vi "RecordFC.vi"(7 "FC-Data":string[][](array[string]), 8 "Latching":bool, 9 "RecordFCdata":bool, 10 "error in (no error)":errorcluster caption="Fehler (Eingang, kein Fehler)", 11 "MultiWii Data Cluster 2":refnum<vi>) -> (2 "error out":errorcluster caption="Fehler (Ausgang)", 5 "FC-Data OUT":string[][](array[string]))   [LabVIEW 2017]
uses:
  IMU_Functions/IMU_Data_Cluster.ctl
  <vilib>/Utility/file.llb/Write To Spreadsheet File (string).vi
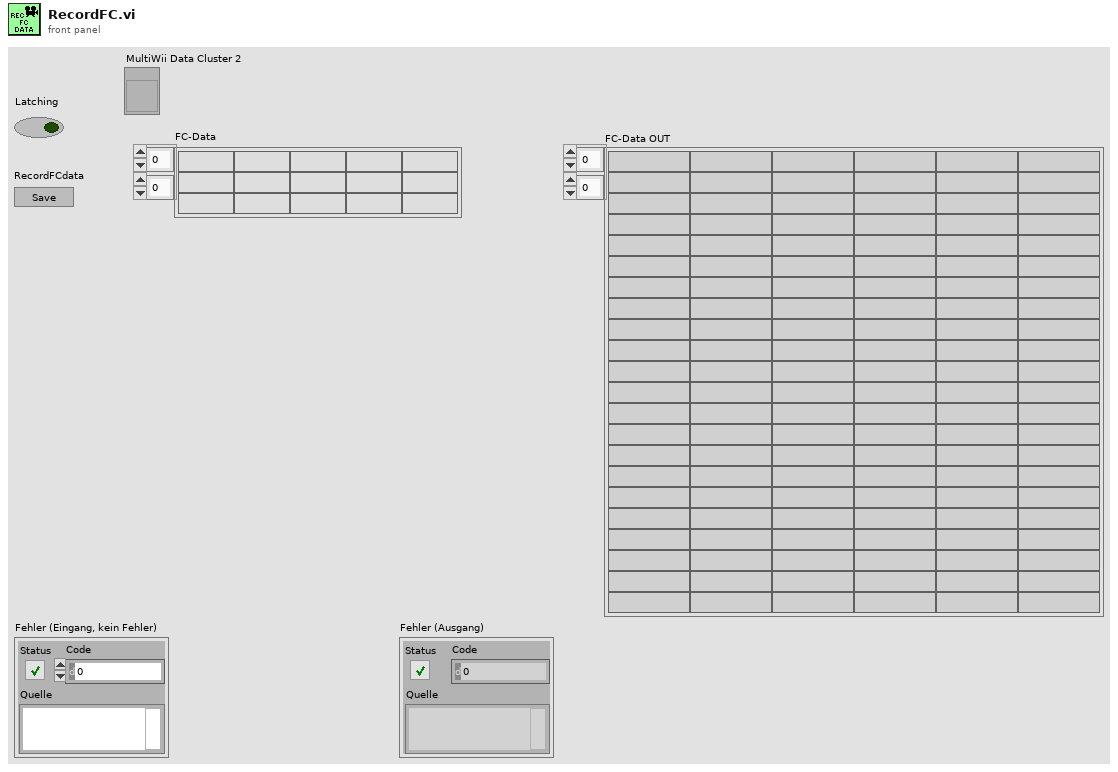
[diagram p1: front panel]
types:
  T1 = typedef "IMU_Data_Cluster.ctl" = cluster{"Firmware Revision":string, "Multitype Name":string, "Cycle Time":u16, "I²C Error Count":u16, "ACC present":bool, "Baro present":bool, "Mag Present":bool, "GPS present":bool, "Sonar present":bool, "Acc X axis (Roll)":dbl, "Acc Y axis (Pitch)":dbl, "Acc Z axis (Yaw)":dbl, "Gyro X axis (Roll)":dbl, "Gyro Y axis (Pitch)":dbl, "Gyro Z axis (Yaw)":dbl, "Mag X axis (Roll)":dbl, "Mag Y axis (Pitch)":dbl, "Mag Z axis (Yaw)":dbl, "X angle (Roll)":dbl, "Y angle (Pitch)":dbl, "Heading [°]":dbl, "Altitude [m]":dbl, "Vario":dbl, "GPS_Fix":u8, "GPS_NumSat":u8, "GPS_coord[LAT]":dbl, "GPS_coord[LON]":dbl, "GPS_Altitude":dbl, "GPS_Speed over Ground":dbl, "GPS_Ground Course":dbl, "Baro P [mbara]":dbl, "Baro T [°C]":dbl, "Altitude abs [m]":dbl}
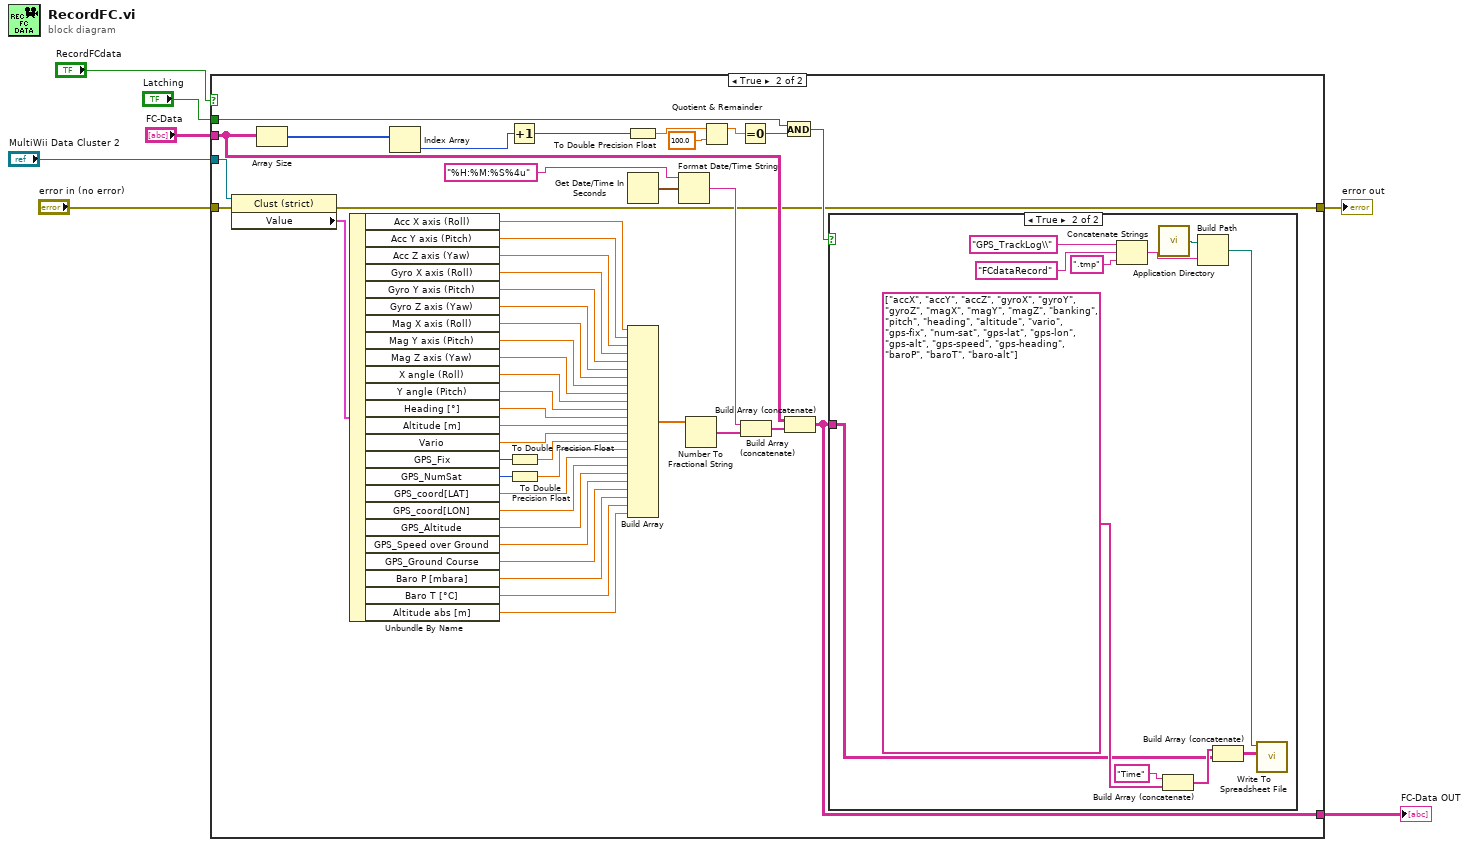
[diagram p0: block diagram]
diagram:
  n1 = case shown="True" "RecordFCdata" {
    tunnel: "FC-Data" -> [w9 w28]
    tunnel: [w9 w22] -> w5
    tunnel: "Latching" -> [_ w20]
    tunnel: "MultiWii Data Cluster 2" -> [_ w13]
    tunnel: "error in (no error)" -> [w8 w11]
    tunnel: [w8 w10] -> w1
    frame False {
    }
    frame True {
      n2 = property class="Clust (strict)"(reference=w13, error in=w11) -> (error out=w10:errorcluster, "Value"=w12:T1)  [unwired: 1 out]
      n3 = Array Size(array=w28) -> (size(s)=w29:i32[])
      n4 = Unbundle By Name(w12) -> ("Acc X axis (Roll)"=w56:dbl, "Acc Y axis (Pitch)"=w55:dbl, "Acc Z axis (Yaw)"=w54:dbl, "Gyro X axis (Roll)"=w53:dbl, "Gyro Y axis (Pitch)"=w52:dbl, "Gyro Z axis (Yaw)"=w51:dbl, "Mag X axis (Roll)"=w50:dbl, "Mag Y axis (Pitch)"=w49:dbl, "Mag Z axis (Yaw)"=w48:dbl, "X angle (Roll)"=w47:dbl, "Y angle (Pitch)"=w46:dbl, "Heading [°]"=w45:dbl, "Altitude [m]"=w43:dbl, "Vario"=w42:dbl, "GPS_Fix"=w41:u8, "GPS_NumSat"=w40:u8, "GPS_coord[LAT]"=w39:dbl, "GPS_coord[LON]"=w38:dbl, "GPS_Altitude"=w37:dbl, "GPS_Speed over Ground"=w36:dbl, "GPS_Ground Course"=w33:dbl, "Baro P [mbara]"=w32:dbl, "Baro T [°C]"=w31:dbl, "Altitude abs [m]"=w30:dbl)
      n5 = Index Array(array=w29) -> (element=w27:i32)  [unwired: 1 in]
      n6 = Increment(x=w27) -> (x+1=w26:i32)
      n7 = To Double Precision Float(number=w41) -> (double precision float=w35:dbl)
      n8 = To Double Precision Float(number=w40) -> (double precision float=w34:dbl)
      n9 = To Double Precision Float(number=w26) -> (double precision float=w23:dbl)
      n10 = Get Date/Time In Seconds() -> (seconds since 1Jan1904=w18:timestamp)
      n11 = Build Array(w56, w55, w54, w53, w52, w51, w50, w49, w48, w47, w46, w45, w43, w42, w35, w34, w39, w38, w37, w36, w33, w32, w31, w30) -> (w44:dbl[])
      n12 = Format Date/Time String(time format string (%c)="%H:%M:%S%4u" ("Zeitformatierungs-String (%c)"), seconds (now)=w18) -> (date/time string=w15:string)  [unwired: 1 in]
      n13 = Number To Fractional String(number=w44) -> (F-format string=w16:string[])  [unwired: 3 in]
      n14 = Quotient & Remainder(x=w23, y=100.0 ("SaveEveryReadings")) -> (x-y*floor(x/y)=w24:dbl)  [unwired: 1 out]
      n15 = Equal To 0?(x=w24) -> (x = 0?=w21:bool)
      n16 = Build Array (concatenate)(w15, w16) -> (w14:string[])
      n17 = And(x=w20, y=w21) -> (x .and. y?=w19:bool)
      n18 = Build Array (concatenate)(w28, w14) -> (w22:string[][])
      n19 = case shown="True" w19 {
        tunnel: w22 -> [_ w64]
        frame False {
        }
        frame True {
          n20 = Concatenate Strings("GPS_TrackLog\\" ("String"), "FCdataRecord" ("String"), ".tmp" ("String")) -> (w61:string)
          n21 = call <vilib>:"Application Directory.vi"() -> ("Application Directory"=w63:path)
          n22 = Build Array (concatenate)("Time", string[] ["accX", "accY", "accZ", "gyroX", "gyroY", "gyroZ", "magX", "magY", "magZ", "banking", "pitch", "heading", "altitude", "vario", "gps-fix", "num-sat", "gps-lat", "gps-lon", "gps-alt", "gps-speed", "gps-heading", "baroP", "baroT", "baro-alt"]) -> (w65:string[])
          n23 = Build Path(base path=w63, name or relative path=w61) -> (appended path=w58:path)
          n24 = Build Array (concatenate)(w65, w64) -> (w59:string[][])
          n25 = call-poly <vilib>:"Write To Spreadsheet File.vi"("2D data"=w59, "file path (dialog if empty)"=w58) -> ()  [unwired: 6 in, 1 out]
        }
      }
    }
  }
  "error out" <- w1
  "FC-Data OUT" <- w5
